vi "onCreated.vi"(8 "error in (no error)":errorcluster, 11 "LIA":refnum<class "LIA.lvclass">) -> (0 "error out":errorcluster, 3 "LIA out":refnum<class "LIA.lvclass">)   [LabVIEW 2017, in "LIA.lvclass"]
doc: "JKI State Machine Objects (SMO) 1.3.0.56\nJKI - JKI\nCopyright (c) 2017, JKI"
uses:
  LIA.lvclass
  D:/Program Files (x86)/National Instruments/LabVIEW 2017/vi.lib/JKI/JKI SMO/SMO/SMO.lvclass
  D:/upwork/Laser Measurement Tool/Laser/project/Subsystems/MeasuringDevice/MeasuringDevice.lvclass
  CircularBuffer/types/type.DBL/type.DBL.lvclass
  D:/upwork/Laser Measurement Tool/Laser/project/Subsystems/CircularBuffer/types/type/type.lvclass
  MeasuringDevice/MeasuringDevice.lvclass
  <vilib>/JKI/JKI SMO/SMO/SMO.lvclass
  CircularBuffer/CircularBuffer.lvclass
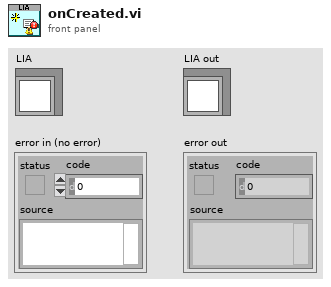
[diagram p1: front panel]
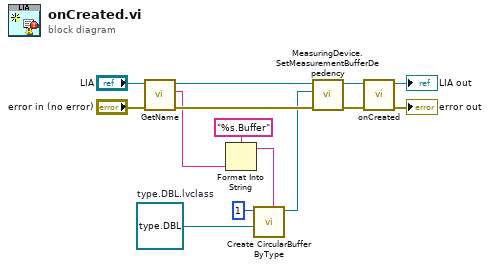
[diagram p0: block diagram]
diagram:
  w11 = refnum<class "type.DBL.lvclass"> refnum  # type.DBL.lvclass
  n1 = call <vilib>:"GetName.vi"("error in (no error)"="error in (no error)", "SMO"="LIA") -> ("error out"=w5:errorcluster, "Name"=w3:string, "SMO out"=w6:refnum<class "LIA.lvclass">)  [unwired: 7 in]
  n2 = Format Into String(format string="%s.Buffer", w3) -> (resulting string=w9:string)  [unwired: 2 in, 1 out]
  n3 = call "Create CircularBuffer ByType.vi"("Buffer Name"=w9, "type"=w11, "BufferSize"=1) -> ("CircularBuffer out"=w4:refnum<class "CircularBuffer.lvclass">)  [unwired: 6 in, 2 out]
  n4 = call "MeasuringDevice.SetMeasurementBufferDepedency.vi"("error in (no error)"=w5, "CircularBuffer"=w4, "MeasuringDevice"=w6) -> ("error out"=w8:errorcluster, "MeasuringDevice"=w7:refnum<class "LIA.lvclass">)  [unwired: 7 in]
  n5 = call-parent "onCreated.vi"("error in (no error)"=w8, "SMO"=w7) -> ("error out"=→"error out":errorcluster, "SMO out"=→"LIA out":refnum<class "LIA.lvclass">)  [unwired: 8 in]
